vi "Open SV Connections.vi"(8 "error in (no error)":errorcluster, 11 "SV B-M (Host) in":refnum<class "SV B-M (Host).lvclass">) -> (0 "error out":errorcluster, 3 "SV B-M (Host) out":refnum<class "SV B-M (Host).lvclass">)   [LabVIEW 2015, in "SV B-M (Host).lvclass"]
doc: "Open connections to all the shared variables that were deployed. Send a command to the target to do the same and wait for acknowledgement that was completed."
uses:
  SV B-M (Host).lvclass
  Type Defs/Stream Param Cluster.ctl
  Type Defs/Sequence Parameters.ctl
  Type Defs/Target Type.ctl
  Type Defs/Variable Data Type.ctl
  SV B-M (Host).lvclass/SV B-M (Host).ctl
  Listbox - In Progress.vi
  Command & Ack - Send Command.vi
  Command & Ack - Receive Ack.vi
  Process Ack Data - Open SVs.vi
  Listbox - Complete.vi
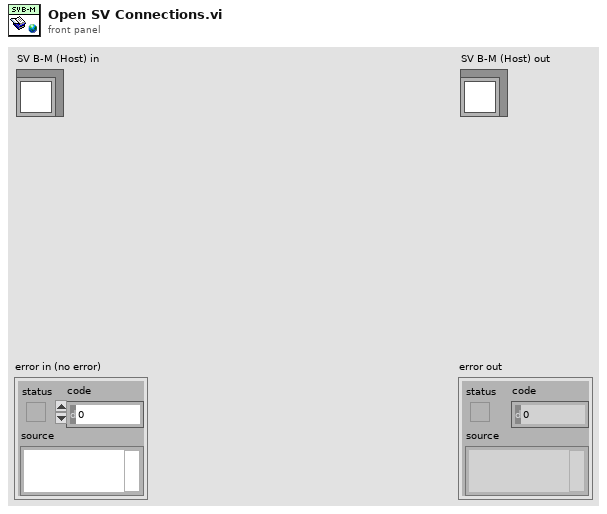
[diagram p1: front panel]
types:
  T1 = typedef "Stream Param Cluster.ctl" = cluster{"Seq Parameters":T2, "SV Library Info":cluster{"Lib Path":path, "Lib Size":u16}[]}
  T2 = typedef "Sequence Parameters.ctl" = cluster{"Test Name":string, "Target":T3, "Host IP Address":string, "Target IP Address":string, "Shared Variable Host":enum16{"Target", "Host"}, "Shared Variable Writer":enum16{"Target", "Host"}, "Variable Data Type":T4, "# of Variables per Library":u16, "Update Rate (Hz)":dbl, "Read Rate (Hz)":dbl, "Floor":u32, "Ceiling":u32, "Delta":u32}
  T3 = typedef "Target Type.ctl" = enum16{"cRIO-9012", "cRIO-9014", "cRIO-9022", "cRIO-9023", "cRIO-9024", "cRIO-9025", "cRIO-9068", "cRIO-9073", "cRIO-9074", "cRIO-9075", "cRIO-9076", "cRIO-9081", "cRIO-9082", "myRIO-1900", "myRIO-1950", "PXI-8101", "PXI-8115", "PXI-8119", "PXI-8820", "PXIe-8100", "PXIe-8101", "PXIe-8133", "PXIe-8135", "PXIe-8820", "sbRIO-9605", "sbRIO-9606", "sbRIO-9623", "sbRIO-9626", "sbRIO-9633", "sbRIO-9636", "Unlisted (Linux-RT)", "Unlisted (PharLap)", "Unlisted (VxWorks)", "Windows Target"}
  T4 = typedef "Variable Data Type.ctl" = enum16{"U8", "U16", "U32", "U64", "I8", "I16", "I32", "I64", "Single", "Double", "Boolean", "String"}
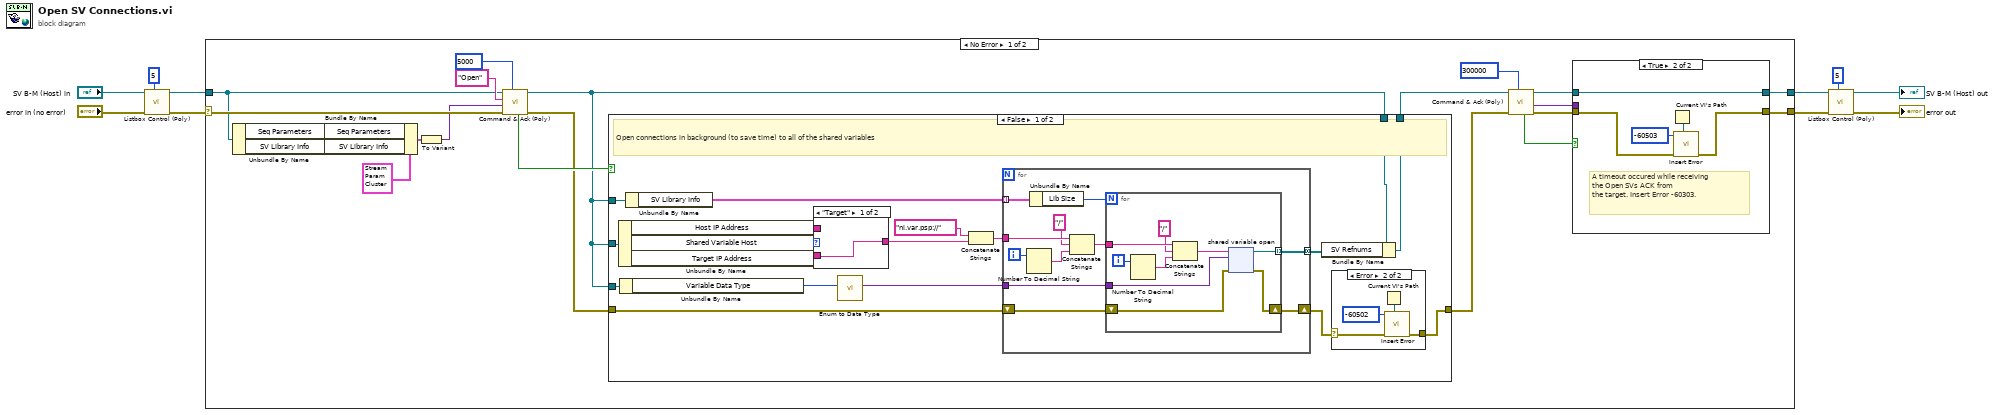
[diagram p0: block diagram]
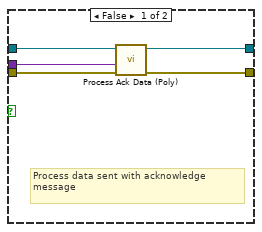
[diagram p2: hidden frame]
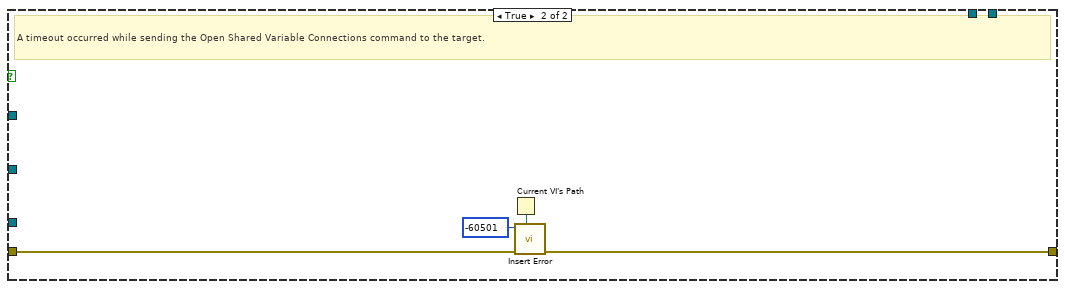
[diagram p5: hidden frame]
diagram:
  n1 = call-poly "Listbox Control (Poly).vi"("Row to Update"=5, "error in (no error)"="error in (no error)", "SV B-M In"="SV B-M (Host) in") -> ("error out"=w7:errorcluster, "SV B-M Out"=w8:refnum<class "SV B-M (Host).lvclass">)  [unwired: 7 in]
  n2 = case shown="No Error" w7 {
    selector: w7 -> [w31 w93]
    tunnel: [w17 w93] -> w3
    tunnel: [w18 w92] -> w4
    tunnel: w8 -> [w15 w92]
    frame No Error {
      n3 = Unbundle By Name(w15) -> ("Seq Parameters"=w14:T2, "SV Library Info"=w13:cluster{"Lib Path":path, "Lib Size":u16}[])
      n4 = Bundle By Name(cluster=T1 {"Seq Parameters"={"Test Name"="Unique Test Name", "Target"=enum."cRIO-9012", "Host IP Address"="0.0.0.0", "Target IP Address"="0.0.0.0", "Shared Variable Host"=enum."Target", "Shared Variable Writer"=enum."Target", "Variable Data Type"=enum."Double", "# of Variables per Library"=500, "Update Rate (Hz)"=1.0, "Read Rate (Hz)"=1.0, "Floor"=500, "Ceiling"=5000, "Delta"=500}, "SV Library Info"=[]} ("Cluster"), "Seq Parameters"=w14, "SV Library Info"=w13) -> (w12:T1)
      n5 = To Variant(anything=w12) -> (Variant=w11:variant)
      n6 = call-poly "Command & Ack (Poly).vi"("Timeout (-1)"=5000, "error in (no error)"=w31, "Message Data"=w11, "Message"="Open", "SV B-M (Host) in"=w15) -> ("error out"=w26:errorcluster, "SV B-M (Host) out"=w25:refnum<class "SV B-M (Host).lvclass">, "Timeout?"=w27:bool)  [unwired: 4 in]
      n7 = case shown="False" w27 {
        tunnel: w26 -> [w44 w91]
        tunnel: w25 -> [w58 _]
        tunnel: [w42 w90] -> w23
        tunnel: w25 -> [w59 _]
        tunnel: w25 -> [w57 _]
        tunnel: w25 -> [w46 w87]
        tunnel: [w45 w87] -> w24
        frame False {
          # "Open connections in background (to save time) to all of the shared variables"
          n8 = Unbundle By Name(w58) -> ("Host IP Address"=w51:string, "Shared Variable Host"=w50:enum16{"Target", "Host"}, "Target IP Address"=w49:string)
          n9 = Unbundle By Name(w57) -> ("Variable Data Type"=w48:T4)
          n10 = Unbundle By Name(w59) -> ("SV Library Info"=w52:cluster{"Lib Path":path, "Lib Size":u16}[])
          n11 = case shown="\"Target\"" w50 {
            tunnel: w51 -> [_ w66]
            tunnel: w49 -> [w65 _]
            tunnel: [w65 w66] -> w53
            frame "Target" {
            }
            frame "Host" {
            }
          }
          n12 = call "Enum to Data Type.vi"("Variable Data Type"=w48) -> ("Variant"=w56:variant)  [unwired: 10 in]
          n13 = Concatenate Strings("ni.var.psp://", w53) -> (w55:string)
          n14 = for {
            tunnel: w52 -> [w77] mode=indexing
            tunnel: w55 -> [w75]
            shift-right: [w67] -> w43
            shift-left: w44 -> [w70]
            tunnel: w56 -> [w69]
            tunnel: [w68] -> w47 mode=concatenating
            i -> [w74]
            n15 = Number To Decimal String(number=w74) -> (decimal integer string=w73:string)  [unwired: 1 in]
            n16 = Unbundle By Name(w77) -> ("Lib Size"=w76:u16)
            n17 = Concatenate Strings(w75, "/", w73) -> (w71:string)
            n18 = for {
              N: w76 -> [_]
              tunnel: w71 -> [w85]
              shift-right: [w79] -> w67
              shift-left: w70 -> [w81]
              tunnel: w69 -> [w80]
              tunnel: [w78] -> w68 mode=indexing
              i -> [w86]
              n19 = Number To Decimal String(number=w86) -> (decimal integer string=w84:string)  [unwired: 1 in]
              n20 = Concatenate Strings(w85, "/", w84) -> (w82:string)
              n21 = shared-variable-open(w82, w81, w80) -> (w78:refnum<k21>, w79:errorcluster)  [unwired: 2 in]
            }
          }
          n22 = Bundle By Name(cluster=w46, "SV Refnums"=w47) -> (w45:refnum<class "SV B-M (Host).lvclass">)
          n23 = case shown="Error" w43 {
            selector: w43 -> [w60 w62]
            tunnel: [w60 w61] -> w42
            frame No Error {
              # "No Error"
            }
            frame Error {
              # "Error while reading / writing from SVs"
              n24 = Current VI's Path() -> (path=w64:path)
              n25 = call "Insert Error.vi"("VI Path"=w64, "error in (no error)"=w62, "Error Code"=-60502) -> ("error out"=w61:errorcluster)  [unwired: 8 in]
            }
          }
        }
        frame True {
          # "A timeout occurred while sending the Open Shared Variable Connections command to the target."
          n26 = Current VI's Path() -> (path=w88:path)
          n27 = call "Insert Error.vi"("VI Path"=w88, "error in (no error)"=w91, "Error Code"=-60501) -> ("error out"=w90:errorcluster)  [unwired: 8 in]
        }
      }
      n28 = call-poly "Command & Ack (Poly).vi"("Timeout (-1)"=300000, "error in (no error)"=w23, "SV B-M (Host) in"=w24) -> ("error out"=w20:errorcluster, "Message Data"=w21:variant, "SV B-M (Host) out"=w22:refnum<class "SV B-M (Host).lvclass">, "Timeout?"=w19:bool)  [unwired: 4 in, 1 out]
      n29 = case shown="True" w19 {
        tunnel: w22 -> [w36 w41]
        tunnel: w20 -> [w34 w40]
        tunnel: [w33 w41] -> w18
        tunnel: [w32 w37] -> w17
        tunnel: w21 -> [w35 _]
        frame False {
          # "Process data sent with acknowledge\nmessage"
          n30 = call-poly "Process Ack Data (Poly).vi"("error in (no error)"=w34, "CPU Load Data"=w35, "SV B-M (Host) in"=w36) -> ("error out"=w32:errorcluster, "SV B-M (Host) out"=w33:refnum<class "SV B-M (Host).lvclass">)  [unwired: 7 in]
        }
        frame True {
          # "A timeout occured while receiving\nthe Open SVs ACK from\nthe target. Insert Error -60303."
          n31 = Current VI's Path() -> (path=w38:path)
          n32 = call "Insert Error.vi"("VI Path"=w38, "error in (no error)"=w40, "Error Code"=-60503) -> ("error out"=w37:errorcluster)  [unwired: 8 in]
        }
      }
    }
    frame Error {
    }
  }
  n33 = call-poly "Listbox Control (Poly).vi"("Row to Update"=5, "error in (no error)"=w3, "SV B-M In"=w4) -> ("error out"=→"error out":errorcluster, "SV B-M Out"=→"SV B-M (Host) out":refnum<class "SV B-M (Host).lvclass">)  [unwired: 7 in]
